vi "Parse design request.vi"(11 "Request":T3={"Key"=["SERVER_PROTOCOL", "SERVER_SOFTWARE", "GATEWAY_INTERFACE", "SERVER_PORT", "SERVER_NAME", "DOCUMENT_ROOT", "SERVER_URL", "SERVER_ADDR", "SERVER_HOST", "QUERY_STRING", "CONTENT_LENGTH", "PATH_INFO", "SCRIPT_FILENAME", "AUTH_TYPE", "REMOTE_HOST", "SERVICE_NAME", "REQUEST_URI", "SERVICE_PATH", "REQUEST_TRANSPORT", "SCRIPT_NAME", "CONTENT_TYPE", "PATH_TRANSLATED", "REMOTE_USER", "REMOTE_ADDR", "REQUEST_METHOD", "CONTENT_LENGTH", "HOST", "CONNECTION", "REFERER", "ACCEPT", "CACHE_CONTROL", "ACCEPT_ENCODING", "CONTENT_TYPE", "ACCEPT_CHARSET", "ACCEPT_LANGUAGE", "USER_AGENT", "ORIGIN", "ProjectCity", "Language", "Q.Plant0.001", "ProjectTitle", "Email", "Name", "countries", "Organization", "ProjectNotes", "ProjectState"], "Value"=[]}) -> (1 "Language":string, 2 "User and project info":T1, 3 "Method":string)   [LabVIEW 2015]
uses:
  RequestKeys.ctl
  Folders.ctl
  Variable cluster.ctl
  user project design.ctl
panel:
  out "Method Found":bool
  out "index of element":i32
  out "FolderPath":path
  out "folder names":string[](array[string])
  out "Design inputs":T1
  in  "datatype":T1
  in  "Request Keys":T2=enum."ProjectNotes"
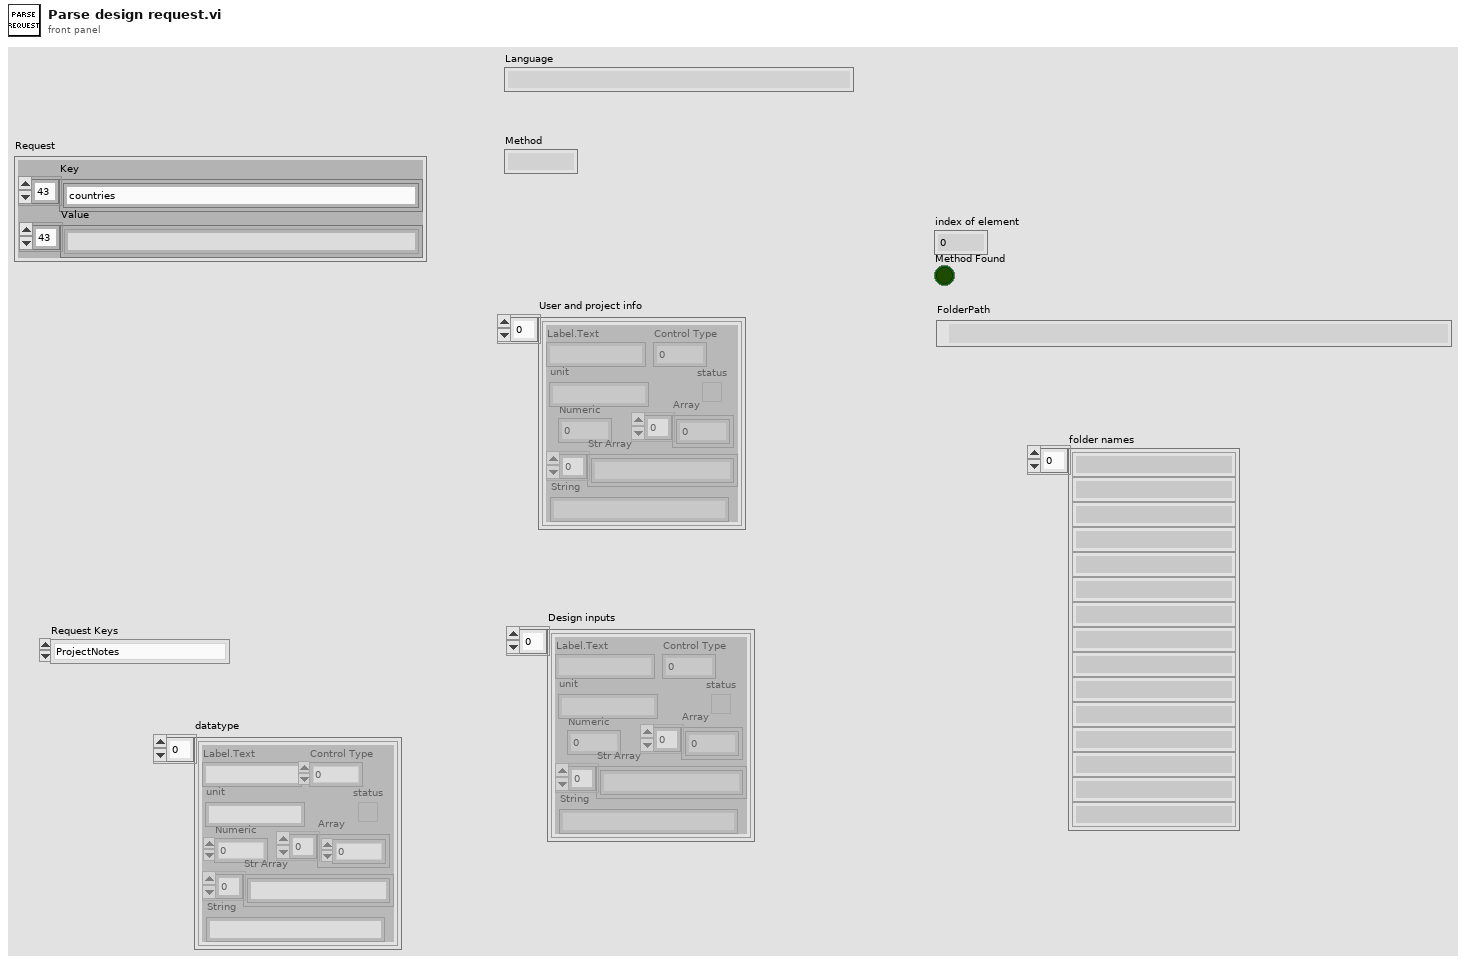
[diagram p1: front panel]
types:
  T1 = typedef "Variable cluster.ctl" = cluster{"Label.Text":string, "Control Type":u32, "Numeric":dbl, "Array":dbl[], "status":bool, "Str Array":string[], "String":string, "unit":string}[]
  T2 = typedef "RequestKeys.ctl" = enum16{"REFERER", "Name", "Email", "Organization", "Language", "Country", "ProjectTitle", "ProjectCity", "ProjectState", "ProjectNotes"}
  T3 = typedef "user project design.ctl" = cluster{"Key":string[], "Value":string[]}
  T4 = typedef "Folders.ctl" = enum16{"DesignTool", "RequestedDesigns", "CompletedDesigns"}
  T5 = cluster{"Label.Text":string, "Control Type":u32, "Numeric":dbl, "Array":dbl[], "status":bool, "Str Array":string[], "String":string, "unit":string}
  T6 = cluster{"Label.Text":string, "Control Type":u32, "Numeric":dbl, "Array":dbl[], "status":bool, "Str Array":string[], "String":string, "unit":string}[]
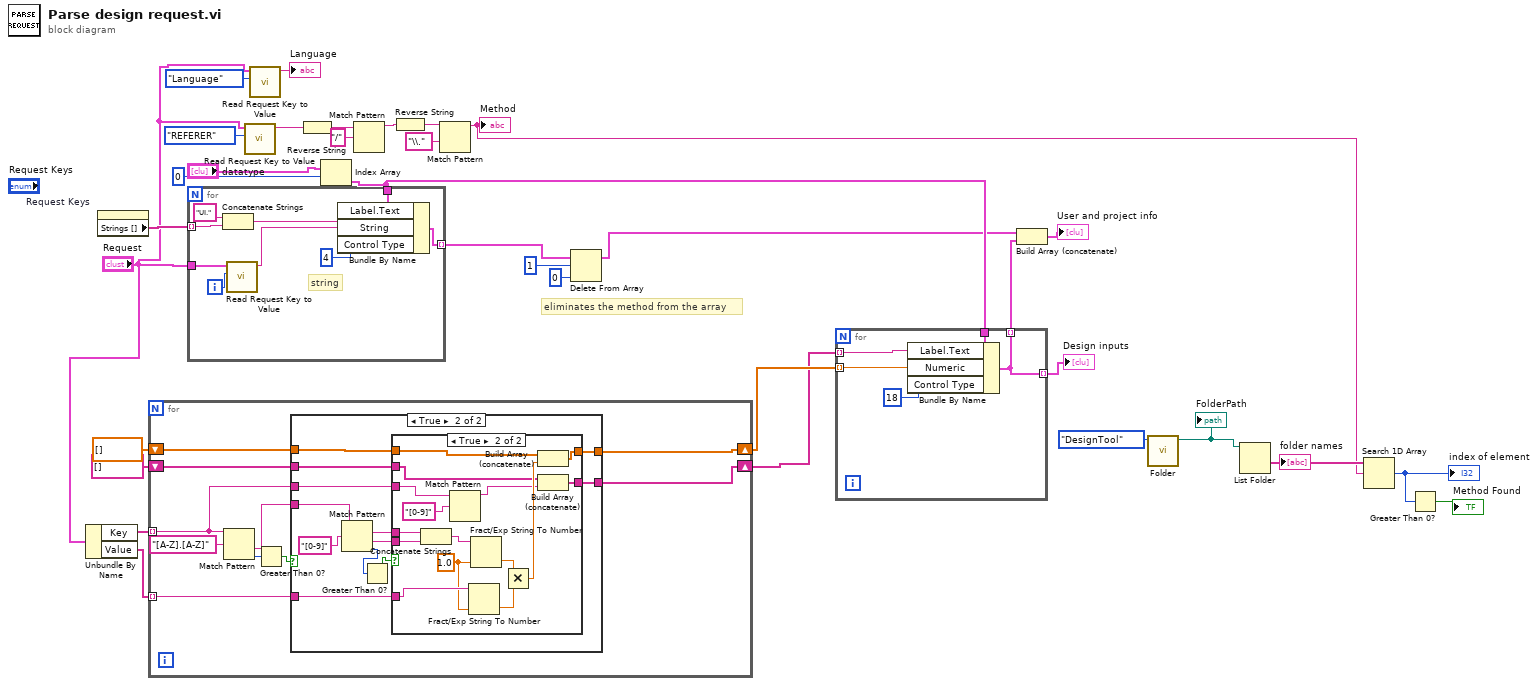
[diagram p0: block diagram]
diagram:
  # "eliminates the method from the array"
  n1 = Unbundle By Name("Request") -> ("Key"=w30:string[], "Value"=w29:string[])
  n2 = property on="Request Keys" class="Enum (strict)"() -> ("Strings []"=w33:string[])  [unwired: 2 in, 2 out]
  n3 = for {
    tunnel: w30 -> [w36] mode=indexing
    shift-right: [w38] -> w25
    shift-left: dbl[] [] -> [w37]
    tunnel: w29 -> [w39] mode=indexing
    shift-right: [w34] -> w24
    shift-left: string[] [] -> [w35]
    n4 = Match Pattern(string=w36, regular expression="[A-Z].[A-Z]") -> (after substring=w40:string, offset past match=w42:i32)  [unwired: 1 in, 2 out]
    n5 = Greater Than 0?(x=w42) -> (x > 0?=w41:bool)
    n6 = case shown="True" w41 {
      tunnel: w40 -> [_ w57]
      tunnel: w39 -> [_ w51]
      tunnel: [w45 w50] -> w38
      tunnel: w37 -> [w45 w49]
      tunnel: w36 -> [_ w48]
      tunnel: w35 -> [w44 w47]
      tunnel: [w44 w46] -> w34
      frame False {
      }
      frame True {
        n7 = Match Pattern(string=w57, regular expression="[0-9]") -> (match substring=w55:string, after substring=w54:string, offset past match=w53:i32)  [unwired: 1 in, 1 out]
        n8 = Greater Than 0?(x=w53) -> (x > 0?=w52:bool)
        n9 = case shown="True" w52 {
          tunnel: w55 -> [_ w74]
          tunnel: w54 -> [_ w73]
          tunnel: w51 -> [_ w72]
          tunnel: [w58 w66] -> w50
          tunnel: w49 -> [w58 w67]
          tunnel: w48 -> [_ w61]
          tunnel: w47 -> [w59 w65]
          tunnel: [w59 w64] -> w46
          frame False {
          }
          frame True {
            w71 = 1.0 ("default (0 DBL)")
            n10 = Concatenate Strings(w74, w73) -> (w63:string)
            n11 = Match Pattern(string=w61, regular expression="[0-9]") -> (before substring=w60:string)  [unwired: 1 in, 3 out]
            n12 = Fract/Exp String To Number(string=w72, default (0 dbl)=w71) -> (number=w70:dbl)  [unwired: 2 in, 1 out]
            n13 = Fract/Exp String To Number(string=w63, default (0 dbl)=w71) -> (number=w69:dbl)  [unwired: 2 in, 1 out]
            n14 = Multiply(x=w69, y=w70) -> (x*y=w68:dbl)
            n15 = Build Array (concatenate)(w67, w68) -> (w66:dbl[])
            n16 = Build Array (concatenate)(w65, w60) -> (w64:string[])
          }
        }
      }
    }
  }
  n17 = call "Read Request Key to Value.vi"("Request Keys"=RequestKeys."REFERER", "Request"="Request") -> ("Value"=w15:string)  [unwired: 9 in]
  n18 = call "Read Request Key to Value.vi"("Request Keys"=RequestKeys."Language", "Request"="Request") -> ("Value"=→"Language":string)  [unwired: 9 in]
  n19 = Reverse String(1:w15) -> (0:w14:string)
  n20 = Index Array(array="datatype", index=0) -> (element=w26:T5)
  n21 = for {
    tunnel: "Request" -> [w83]
    tunnel: w33 -> [w81] mode=indexing
    tunnel: [w80] -> w17 mode=indexing
    tunnel: w26 -> [w77]
    i -> [w82]
    # "string"
    n22 = Concatenate Strings("UI." ("string"), w81) -> (w79:string)
    n23 = call "Read Request Key to Value.vi"("Request Keys"=w82, "Request"=w83) -> ("Value"=w76:string)  [unwired: 9 in]
    n24 = Bundle By Name(cluster=w77, "Label.Text"=w79, "String"=w76, "Control Type"=u32 4) -> (w80:T5)
  }
  n25 = Match Pattern(string=w14, regular expression="/") -> (before substring=w12:string)  [unwired: 1 in, 3 out]
  n26 = Reverse String(1:w12) -> (0:w11:string)
  n27 = Match Pattern(string=w11, regular expression="\\.") -> (before substring=w4:string)  [unwired: 1 in, 3 out]
  "Method" <- w4
  n28 = Delete From Array(array=w17, length=1, index=0) -> (array with subset deleted=w16:T6)  [unwired: 1 out]
  n29 = for {
    tunnel: w26 -> [w88]
    tunnel: w25 -> [w86] mode=indexing
    tunnel: w24 -> [w85] mode=indexing
    tunnel: [w84] -> w22 mode=indexing
    tunnel: [w84] -> w21 mode=indexing
    n30 = Bundle By Name(cluster=w88, "Label.Text"=w85, "Numeric"=w86, "Control Type"=u32 18) -> (w84:T5)
  }
  "Design inputs" <- w21
  n31 = Build Array (concatenate)(w16, w22) -> (→"User and project info":T6)
  n32 = call "Folder.vi"("Folders"=Folders."DesignTool") -> ("FolderPath"=w8:path)  [unwired: 9 in, 1 out]
  "FolderPath" <- w8
  n33 = List Folder(path=w8) -> (folder names=w7:string[])  [unwired: 3 in, 3 out]
  "folder names" <- w7
  n34 = Search 1D Array(1D array=w7, element=w4) -> (index of element=w6:i32)  [unwired: 1 in]
  "index of element" <- w6
  n35 = Greater Than 0?(x=w6) -> (x > 0?=→"Method Found":bool)
